vi "Update Database.vi"(8 "error in (no error)":errorcluster, 11 "Module in":refnum<class "Module.lvclass">) -> (0 "error out":errorcluster, 3 "Module out":refnum<class "Module.lvclass">)   [LabVIEW 2016, in "Module.lvclass"]
uses:
  Module.lvclass
  Module.lvclass/Module.ctl
  <vilib>/drjdpowell/SQLite Library/SQL Statement/SQL Statement.lvclass/SQL Statement.ctl
  <vilib>/drjdpowell/SQLite Library/SQL Connection/Open (string).vi
  <vilib>/drjdpowell/SQLite Library/SQL Statement/Bind Real.vi
  <vilib>/drjdpowell/SQLite Library/SQL Statement/Step.vi
  <vilib>/drjdpowell/SQLite Library/SQL Connection/Execute SQL (No results).vi
  <vilib>/drjdpowell/SQLite Library/SQL Statement/Error Message.vi
  <vilib>/drjdpowell/SQLite Library/SQL Connection/Connection.lvclass
  <vilib>/drjdpowell/SQLite Library/SQL Statement/SQL Statement.lvclass
  <vilib>/drjdpowell/SQLite Library/Transaction Helpers/Transaction.lvlib
  <vilib>/drjdpowell/SQLite Library/SQLite.lvlib
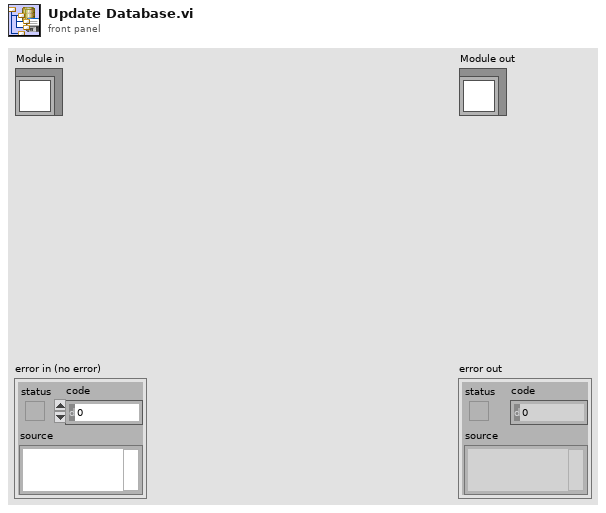
[diagram p1: front panel]
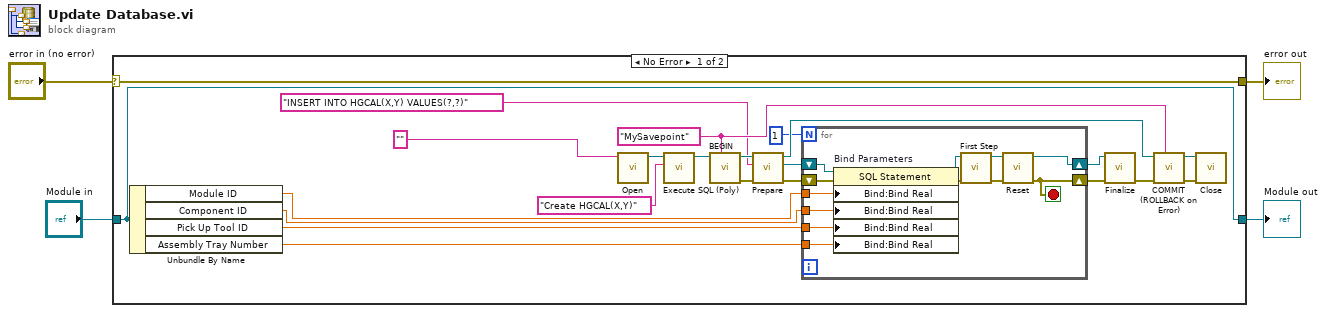
[diagram p0: block diagram]
diagram:
  n1 = case shown="No Error" "error in (no error)" {
    selector: "error in (no error)" -> [w27 w41]
    tunnel: [w27 w41] -> w3
    tunnel: [w15 w40] -> w1
    tunnel: "Module in" -> [w15 w40]
    frame No Error {
      w24 = "MySavepoint" ("Savepoint name")
      n2 = Unbundle By Name(w15) -> ("Module ID"=w8:dbl, "Component ID"=w11:dbl, "Pick Up Tool ID"=w12:dbl, "Assembly Tray Number"=w10:dbl)
      n3 = call-poly <vilib>:"Open.vi"("db file"="") -> ("SQLite Connection"=w7:refnum<class "Connection.lvclass">)  [unwired: 9 in, 1 out]
      n4 = call-poly <vilib>:"Execute SQL (Poly).vi"("SQL"="Create HGCAL(X,Y)", "SQLite Connection in"=w7) -> ("SQLite Connection"=w6:refnum<class "Connection.lvclass">)  [unwired: 8 in, 1 out]
      n5 = call <vilib>:"BEGIN.vi"("Savepoint name"=w24, "SQLite Connection in"=w6) -> ("error out"=w23:errorcluster, "SQLite Connection"=w22:refnum<class "Connection.lvclass">)  [unwired: 8 in]
      n6 = call <vilib>:"Prepare.vi"("error in (no error)"=w23, "SQL"="INSERT INTO HGCAL(X,Y) VALUES(?,?)", "SQLite Connection in"=w22) -> ("error out"=w18:errorcluster, "SQL Statement"=w17:refnum<class "SQL Statement.lvclass">, "SQLite Connection"=w25:refnum<class "Connection.lvclass">)  [unwired: 4 in, 2 out]
      n7 = for {
        N: 1 -> [_]
        shift-right: [w33] -> w20
        shift-left: w17 -> [w39]
        shift-right: [w32] -> w21
        shift-left: w18 -> [w36]
        tunnel: w8 -> [w31]
        tunnel: w12 -> [w30]
        tunnel: w11 -> [w29]
        tunnel: w10 -> [w28]
        stop <- w32 stop-if-true
        n8 = property on="Bind Parameters" class="SQL Statement"(reference=w39, error in=w36, "Bind:Bind Real"=w31, "Bind:Bind Real"=w29, "Bind:Bind Real"=w30, "Bind:Bind Real"=w28) -> (reference out=w38:refnum<class "SQL Statement.lvclass">, error out=w37:errorcluster)
        n9 = call <vilib>:"First Step.vi"("error in (no error)"=w37, "SQL Statement in"=w38) -> ("error out"=w35:errorcluster, "SQL Statement"=w34:refnum<class "SQL Statement.lvclass">)  [unwired: 7 in, 1 out]
        n10 = call <vilib>:"Reset.vi"("error in (no error)"=w35, "SQL Statement in"=w34) -> ("error out"=w32:errorcluster, "SQL Statement"=w33:refnum<class "SQL Statement.lvclass">)  [unwired: 8 in]
      }
      n11 = call <vilib>:"Finalize.vi"("error in (no error)"=w21, "SQL Statement in"=w20) -> ("error out"=w26:errorcluster)  [unwired: 9 in]
      n12 = call <vilib>:"COMMIT (ROLLBACK on Error).vi"("Savepoint name"=w24, "error in (no error)"=w26, "SQLite Connection in"=w25) -> ("error out"=w13:errorcluster, "SQLite Connection"=w14:refnum<class "Connection.lvclass">)  [unwired: 7 in]
      n13 = call-dynamic "Close.vi"("error in (no error)"=w13, "SQLite Connection in"=w14) -> ()  [unwired: 9 in, 1 out]
    }
    frame Error {
    }
  }
  "error out" <- w3
  "Module out" <- w1
